vi "Launch Root Model.vi"(8 "error in (no error)":errorcluster, 11 "IViewModel In":refnum<class "IViewModel.lvclass">) -> (0 "error out":errorcluster, 3 "IViewModel Out":refnum<class "IViewModel.lvclass">)   [LabVIEW 2017, in "IViewModel.lvlib" / "IViewModel.lvclass"]
doc: "<License>\nCopyright © 2017 Composed Systems, LLC | All rights reserved\nwww.composed.io\n\nAuthor: Ethan Stern <ethan.stern@composed.io>\n\nThis software is provided \"AS IS\" WITHOUT WARRANTIES, either express or implied, AND IS FOR EDUCATIONAL PURPOSES ONLY.\n</License>"
uses:
  <vilib>/gpm_packages/@cs/mva-viewable/Source/IViewModel/IViewModel/IViewModel.lvclass
  C:/Program Files/National Instruments/LabVIEW 2017/vi.lib/ActorFramework/Actor/Actor.lvclass
  C:/Program Files/National Instruments/LabVIEW 2017/vi.lib/gpm_packages/@cs/mva-core/Source/IObserver/IObserver/IObserver.lvclass
  <vilib>/gpm_packages/@cs/mva-viewable/Source/IViewModel/IViewModel/IViewModel.lvclass/IViewModel.ctl
  <vilib>/gpm_packages/@cs/mva-core/Source/IModel/IModel/IModel.lvclass/IModel.ctl
  <vilib>/gpm_packages/@cs/mva-core/Source/IObserver/IObserver/IObserver.lvclass/IObserver.ctl
  <vilib>/gpm_packages/@cs/mva-core/Source/IMediator/IMediator/IMediator.lvclass
  <vilib>/gpm_packages/@cs/mva-core/Source/IModel/IModel/IModel.lvclass
  <vilib>/ActorFramework/Actor/Actor.lvclass
  <vilib>/gpm_packages/@cs/mva-core/Source/IObserver/IObserver/IObserver.lvclass
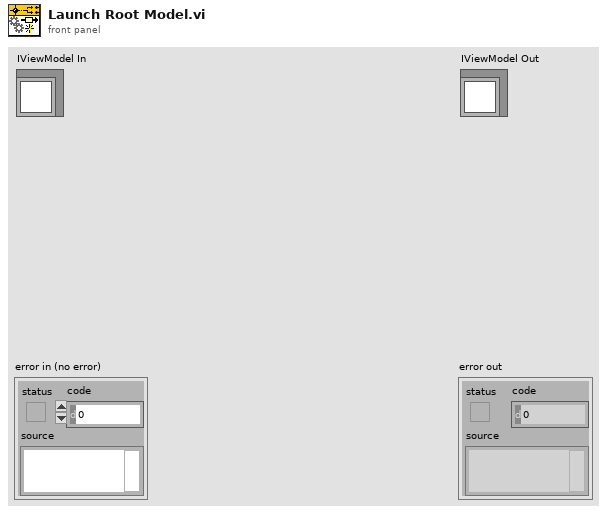
[diagram p1: front panel]
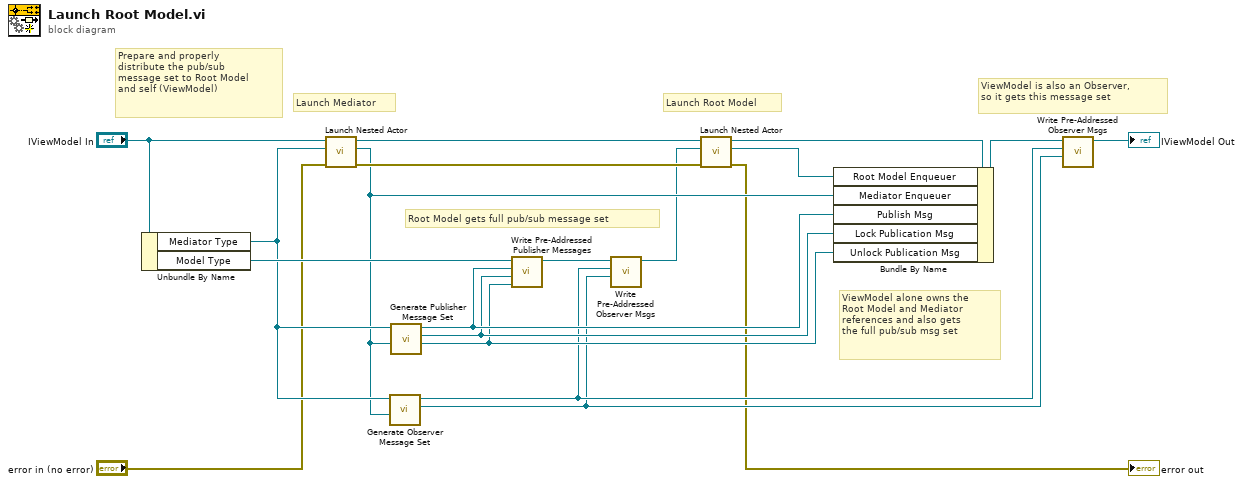
[diagram p0: block diagram]
diagram:
  # "ViewModel is also an Observer,\nso it gets this message set"
  # "Root Model gets full pub/sub message set"
  # "Prepare and properly\ndistribute the pub/sub\nmessage set to Root Model\nand self (ViewModel)"
  # "Launch Root Model"
  # "Launch Mediator"
  # "ViewModel alone owns the\nRoot Model and Mediator\nreferences and also gets\nthe full pub/sub msg set"
  n1 = Unbundle By Name("IViewModel In") -> ("Mediator Type"=w10:refnum<class "IMediator.lvclass">, "Model Type"=w17:refnum<class "IModel.lvclass">)
  n2 = call <vilib>:"Launch Nested Actor.vi"("error in (no error)"="error in (no error)", "Nested Actor"=w10, "Caller Actor in"="IViewModel In") -> ("error out"=w13:errorcluster, "Nested Actor's Enqueuer"=w9:refnum<class "Message Enqueuer.lvclass">, "Caller Actor out"=w18:refnum<class "IViewModel.lvclass">)  [unwired: 6 in]
  n3 = call-dynamic "Generate Observer Message Set.vi"("Mediator Enqueuer"=w9, "Mediator Type"=w10) -> ("Unsubscribe Msg"=w4:refnum<class "Unsubscribe Msg.lvclass">, "Subscribe Msg"=w5:refnum<class "Subscribe Msg.lvclass">)  [unwired: 8 in]
  n4 = call-dynamic "Generate Publisher Message Set.vi"("Mediator Enqueuer"=w9, "IMediator in"=w10) -> ("Unlock Publication Msg"=w6:refnum<class "Unlock Publication Msg.lvclass">, "Lock Publication Msg"=w7:refnum<class "Lock Publication Msg.lvclass">, "Publish Msg"=w8:refnum<class "Publish Msg.lvclass">)  [unwired: 7 in]
  n5 = call <vilib>:"Write Pre-Addressed Publisher Messages.vi"("Pre-Addressed Unlock Publication Msg"=w6, "Pre-Addressed Lock Publication Msg"=w7, "Pre-Addressed Publish Msg"=w8, "IModel in"=w17) -> ("IModel out"=w12:refnum<class "IModel.lvclass">)  [unwired: 7 in]
  n6 = call <vilib>:"Write Pre-Addressed Observer Msgs.vi"("Pre-Addressed Unsubscribe Msg"=w4, "Pre-Addressed Subscribe Msg"=w5, "IObserver In"=w12) -> ("IObserver Out"=w1:refnum<class "IModel.lvclass">)  [unwired: 8 in]
  n7 = call <vilib>:"Launch Nested Actor.vi"("error in (no error)"=w13, "Nested Actor"=w1, "Caller Actor in"=w18) -> ("error out"=→"error out":errorcluster, "Nested Actor's Enqueuer"=w14:refnum<class "Message Enqueuer.lvclass">, "Caller Actor out"=w16:refnum<class "IViewModel.lvclass">)  [unwired: 6 in]
  n8 = Bundle By Name(cluster=w16, "Root Model Enqueuer"=w14, "Mediator Enqueuer"=w9, "Publish Msg"=w8, "Lock Publication Msg"=w7, "Unlock Publication Msg"=w6) -> (w15:refnum<class "IViewModel.lvclass">)
  n9 = call <vilib>:"Write Pre-Addressed Observer Msgs.vi"("Pre-Addressed Unsubscribe Msg"=w4, "Pre-Addressed Subscribe Msg"=w5, "IObserver In"=w15) -> ("IObserver Out"=→"IViewModel Out":refnum<class "IViewModel.lvclass">)  [unwired: 8 in]
